vi "Configure.vi"(8 "error in (no error)":errorcluster, 10 "Digital Configuration Parameters":T1) -> (0 "error out":errorcluster, 3 "Mech Pump out":refnum<class "Mech Pump.lvclass">)   [LabVIEW 2021, in "Mech Pump.lvclass"]
uses:
  Mech Pump.lvclass
  <vilib>/NathanCo/Digital-Tasks/Utilities/Digital Configuration Parameters.ctl
  Mech Pump.lvclass/Mech Pump.ctl
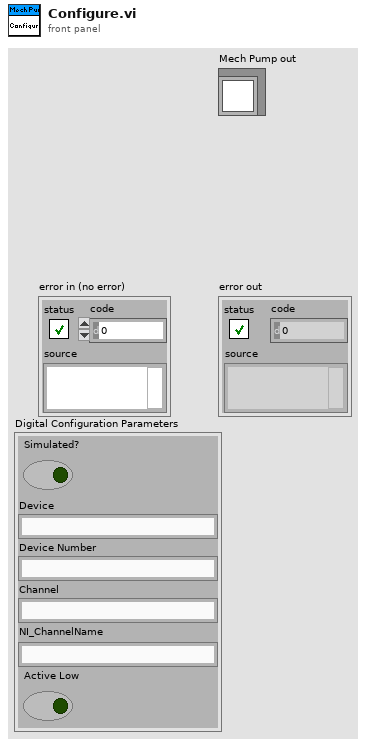
[diagram p1: front panel]
types:
  T1 = typedef "Digital Configuration Parameters.ctl" = cluster{"Simulated?":bool, "Device":string, "Device Number":string, "Channel":string, "NI_ChannelName":string, "Active Low":bool}
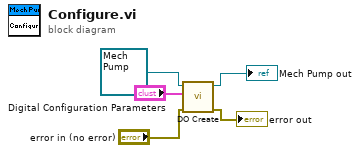
[diagram p0: block diagram]
diagram:
  n1 = call "DO Create.vi"("error in (no error)"="error in (no error)", "Digital Configuration Parameters"="Digital Configuration Parameters", "Mech Pump in"=refnum<class "Mech Pump.lvclass"> refnum) -> ("error out"=→"error out":errorcluster, "Mech Pump out"=→"Mech Pump out":refnum<class "Mech Pump.lvclass">)  [unwired: 7 in]
